vi "Common_Py_Get_Error.vi"(0 "session in":refnum<k35>, 5 "module path":path=path "D:/dev/Guy_Storage/Work/Cancun/MW_Display_Test/Magewell Capture/Capture_LV.py", 11 "error in":errorcluster) -> (4 "session out":refnum<k35>, 6 "module path out":path, 14 "Error Message":string, 15 "error out":errorcluster)   [LabVIEW 2023]
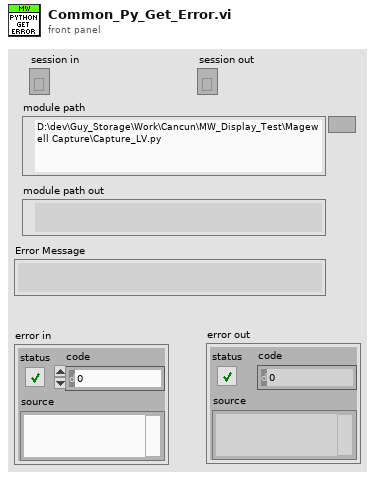
[diagram p1: front panel]
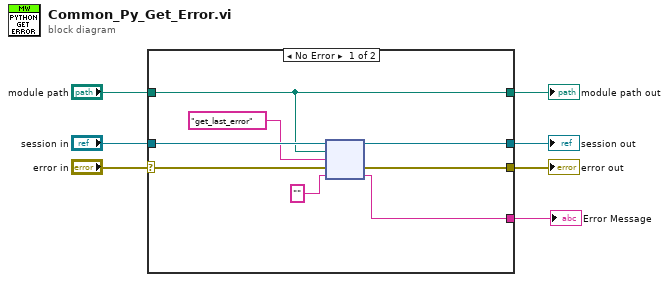
[diagram p0: block diagram]
diagram:
  n1 = case shown="No Error" "error in" {
    selector: "error in" -> [w12 w17]
    tunnel: "module path" -> [w10 w16]
    tunnel: "session in" -> [w15 w18]
    tunnel: [w14 w17] -> w3
    tunnel: [w13 w18] -> w5
    tunnel: [w10 w16] -> w2
    tunnel: [w8 _] -> w1
    frame No Error {
      n2 = node(w15, w10, "get_last_error" ("function name"), w12, "") -> (w13:refnum<k35>, w14:errorcluster, w8:string)  [unwired: 2 out]
    }
    frame Error {
    }
  }
  "session out" <- w5
  "error out" <- w3
  "module path out" <- w2
  "Error Message" <- w1
